vi "FPGAcode4_Debug.vi"() -> ()   [LabVIEW 2015]
uses:
  Limits_In.ctl
  Discard_Points.ctl
  Filter_Cluster.ctl
  <vilib>/Platform/TimedLoop/XDataNode/timing_clust.ctl
  <vilib>/Platform/TimedLoop/XDataNode/nitl_modes.ctl
  <vilib>/Platform/TimedLoop/XDataNode/wakeup.ctl
  Detector_Cluster.ctl
  Correlations.ctl
  <vilib>/rvi/Emulation/niFpgaGetClockAttributes.vi
  <vilib>/rvi/Emulation/niFpgaSctlEmulationGetInTimedLoop.vi
  <vilib>/rvi/Emulation/niFpgaEmulationReportErrorSimple.vi
  <vilib>/rvi/Emulation/niFpgaProcessEmulError.vi
  <vilib>/rvi/eio/common/nirviEmuTemplateMethod_errors.vi
  <vilib>/rvi/Emulation/niFpgaCriticalErrorInLSC.vi
  <vilib>/eio/EIONode/EIONode.xnode
  <vilib>/Platform/TimedLoop/XDataNode/XDataNode.xnode
  <vilib>/Platform/TimedLoop/XDataNode/XDNodeRunTimeDep.lvlib
panel:
  in  "User Trigger?":bool
  out "Charge":T1
  out "Mass":T2
  out "Velocity Count":T3
  in  "User Trigger Distance":fxp<+/-,34,18> format="%.3g"
  out "User Trigger":bool
  out "Particles Discarded":i16
  out "All Discard Points":T4
  in  "Boxcar 3 Size Factor":fxp<+/-,32,16>=0.1999969482421875 format="%.2g"
  in  "Charge Error Factor":fxp<+/-,32,16>=1.100006103515625 format="%.2g"
  in  "Max Correlation Factor":fxp<+,32,4>=0.25 format="%.3g"
  in  "Threshold Factor":fxp<+/-,32,16>=1.0 format="%.2g"
  out "DCS 2":bool
  out "Detectors":cluster{"Det 1":i16, "Det 3":i16}
  out "DCS 1":bool
  in  "Limits":T6
  in  "Calibrate":bool=TRUE
  in  "Armed":bool
  out "Plates":bool
  in  "One Shot":bool
  # "These factors above are in the front\npanel so it is possible to experiment\nwith many different configurations\nof the FPGA on the fly. One can even\nchange the relative size of one filter."
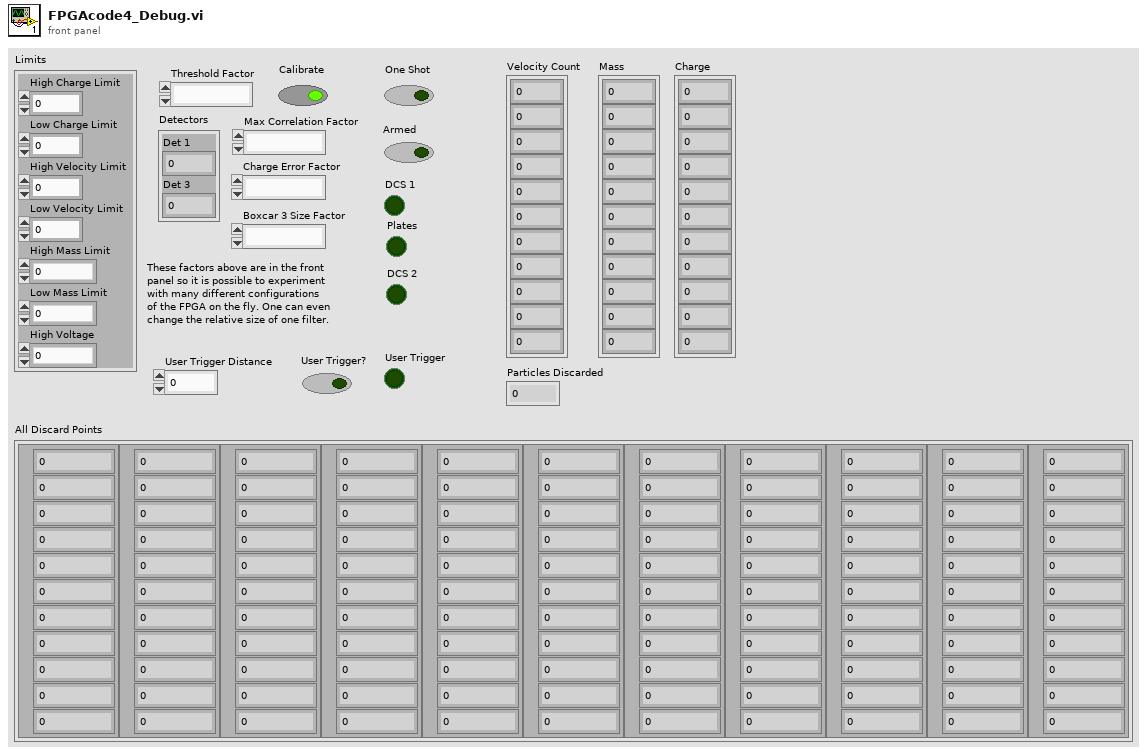
[diagram p1: front panel]
types:
  T1 = cluster{"[0]":fxp<+/-,64,-10>, "[1]":fxp<+/-,64,-10>, "[2]":fxp<+/-,64,-10>, "[3]":fxp<+/-,64,-10>, "[4]":fxp<+/-,64,-10>, "[5]":fxp<+/-,64,-10>, "[6]":fxp<+/-,64,-10>, "[7]":fxp<+/-,64,-10>, "[8]":fxp<+/-,64,-10>, "[9]":fxp<+/-,64,-10>, "[10]":fxp<+/-,64,-10>}
  T2 = cluster{"[0]":fxp<+/-,64,-2>, "[1]":fxp<+/-,64,-2>, "[2]":fxp<+/-,64,-2>, "[3]":fxp<+/-,64,-2>, "[4]":fxp<+/-,64,-2>, "[5]":fxp<+/-,64,-2>, "[6]":fxp<+/-,64,-2>, "[7]":fxp<+/-,64,-2>, "[8]":fxp<+/-,64,-2>, "[9]":fxp<+/-,64,-2>, "[10]":fxp<+/-,64,-2>}
  T3 = cluster{"[0]":i32, "[1]":i32, "[2]":i32, "[3]":i32, "[4]":i32, "[5]":i32, "[6]":i32, "[7]":i32, "[8]":i32, "[9]":i32, "[10]":i32}
  T4 = typedef "Discard_Points.ctl" = cluster{"Discard Points 1":T5, "Discard Points 2":T5, "Discard Points 3":T5, "Discard Points 4":T5, "Discard Points 5":T5, "Discard Points 6":T5, "Discard Points 7":T5, "Discard Points 8":T5, "Discard Points 9":T5, "Discard Points 10":T5, "Discard Points 11":T5}
  T5 = typedef "Filter_Cluster.ctl" = cluster{"1":i32, "2":i32, "3":i32, "4":i32, "5":i32, "6":i32, "7":i32, "8":i32, "9":i32, "10":i32, "11":i32}
  T6 = typedef "Limits_In.ctl" = cluster{"High Charge Limit":fxp<+,32,-41>, "Low Charge Limit":fxp<+,32,-41>, "High Velocity Limit":fxp<+,18,18>, "Low Velocity Limit":fxp<+,18,18>, "High Mass Limit":fxp<+/-,33,-35>, "Low Mass Limit":fxp<+/-,33,-35>, "High Voltage":fxp<+,16,22>}
  T7 = typedef "Detector_Cluster.ctl" = cluster{"Det 1":i32, "Det 2":i32}
  T8 = cluster{"Filter 1":T7, "Filter 2":T7, "Filter 3":T7, "Filter 4":T7}
  T9 = cluster{"Distance to PSU":fxp<+/-,32,5>, "Distance to end of PSU":fxp<+/-,32,5>, "Distance to DCS 2":fxp<+/-,32,5>, "Distance to DCS 1":fxp<+/-,32,5>, "Distance to front of LEIL Chamber":fxp<+/-,32,5>}
  T10 = cluster{"Detector Max Speed Count":i32, "Detector Min Speed Count":i32, "Gap Max Speed Count":i32, "Gap Min Speed Count":i32}
  T11 = cluster{"Distance to PSU":fxp<+/-,64,22>, "Distance to end of PSU":fxp<+/-,64,22>, "Distance to DCS 2":fxp<+/-,64,22>, "Distance to DCS 1":fxp<+/-,64,22>, "Distance to front of LEIL Chamber":fxp<+/-,64,22>}
  T12 = typedef "XDNodeRunTimeDep.lvlib/timing_clust.ctl" = cluster{"Expected End [f-1]":u64, "Actual End [f-1]":u64, "Finished Late? [f-1]":bool, "Expected End [i-1]":u64, "Actual End [i-1]":u64, "Finished Late? [i-1]":bool, "Expected Start [i]":u64, "Actual Start [i]":u64, "Expected Start [f]":u64, "Actual Start [f]":u64, "Source Name":string, "Structure Name":string, "Period":i64, "Deadline":i64, "Offset":i64, "Start":i64, "Priority":i32, "Timeout":i32, "Mode":T13, "Wakeup Reason":T14, "Error":errorcluster, "Source Type":string, "Secondary Source Type":string, "Global End Time":u64, "Global Start Time":u64, "Frame Duration":u64, "Iteration Duration":u64, "Assigned CPU":i32, "I/O Scan Engine Mode":u32}
  T13 = typedef "XDNodeRunTimeDep.lvlib/nitl_modes.ctl" = enum32{"No Change", "Process missed periods, maintain original phase", "Discard missed periods, maintain original phase", "Process missed periods, ignore original phase", "Discard missed periods, ignore original phase"}
  T14 = typedef "XDNodeRunTimeDep.lvlib/wakeup.ctl" = enum32{"Normal", "Aborted", "Asynchronous wakeup", "Timing source error", "Timed loop error", "Timeout"}
  T15 = cluster{"Filter 1":T7, "Filter 2":T7, "Filter 3":T7, "Filter 4":T7}[]
  T16 = cluster{"First Detector Count":i32, "Detector Gap Count":i32, "Second Detector Count":i32, "Second Detector Final Count":i32}
  T17 = typedef "Correlations.ctl" = cluster{"First Correlation":i32, "Latest Correlation":i32}
  T18 = cluster{"Detectors":cluster{"Det 1":i16, "Det 3":i16}, cluster{"Det 1":i16, "Det 2":i16}, cluster{"Det 1":i16, "Det 2":i16}, cluster{"Det 1":i16, "Det 2":i16}}
  T19 = cluster{cluster{"Det 1":i16, "Det 2":i16}, cluster{"Det 1":i16, "Det 2":i16}, cluster{"Det 1":i16, "Det 2":i16}, cluster{"Det 1":i16, "Det 2":i16}}
  T20 = cluster{"Distance to PSU":fxp<+/-,64,54>, "Distance to end of PSU":fxp<+/-,64,54>, "Distance to DCS 2":fxp<+/-,64,54>, "Distance to DCS 1":fxp<+/-,64,54>, "Distance to front of LEIL Chamber":fxp<+/-,64,54>}
  T21 = cluster{"Distance to PSU":i32, "Distance to end of PSU":i32, "Distance to DCS 2":i32, "Distance to DCS 1":i32, "Distance to front of LEIL Chamber":i32}
  T22 = cluster{"[0]":u8, "[1]":u8, "[2]":u8, "[3]":u8, "[4]":u8, "[5]":u8, "[6]":u8, "[7]":u8, "[8]":u8, "[9]":u8, "[10]":u8}
  T23 = cluster{"All Discard Points[0]":T5, "All Discard Points[1]":T5, "All Discard Points[2]":T5, "All Discard Points[3]":T5, "All Discard Points[4]":T5, "All Discard Points[5]":T5, "All Discard Points[6]":T5, "All Discard Points[7]":T5, "All Discard Points[8]":T5, "All Discard Points[9]":T5, "All Discard Points[10]":T5}
  T24 = cluster{i32[], fxp<+/-,64,-2>[], fxp<+/-,64,-10>[]}
  T25 = cluster{"IO Module\\AI 0":i16, "IO Module\\AI 1":i16}
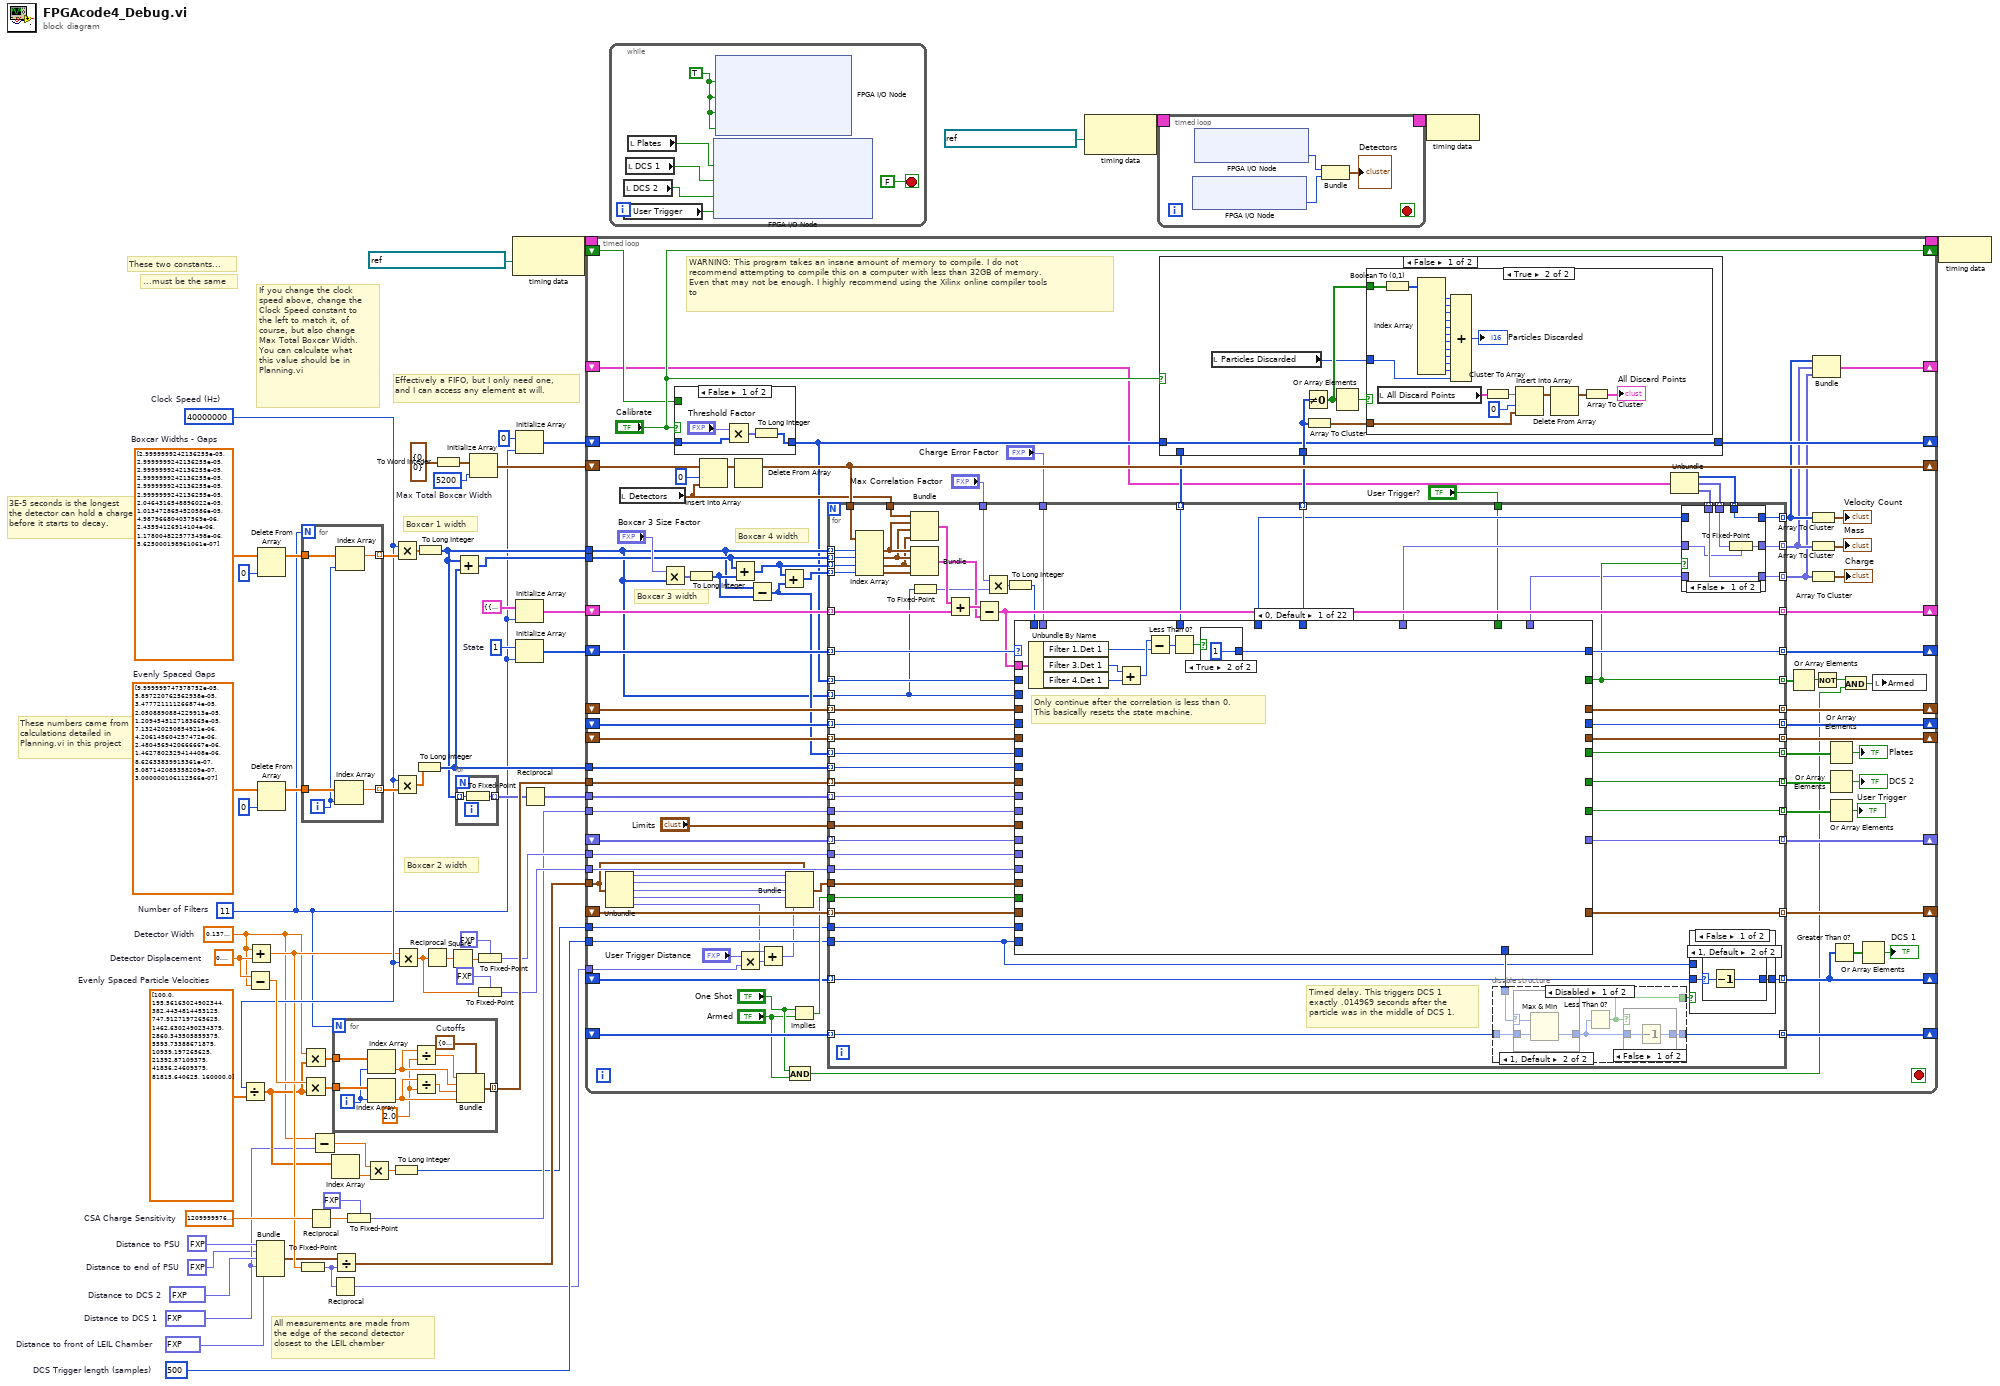
[diagram p0: block diagram]
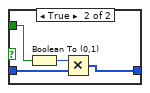
[diagram p2: hidden frame]
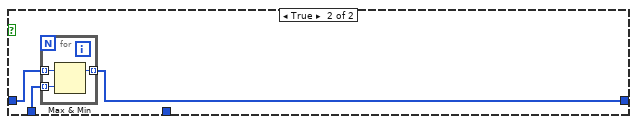
[diagram p4: hidden frame]
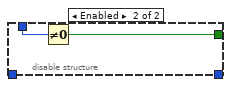
[diagram p10: hidden frame]
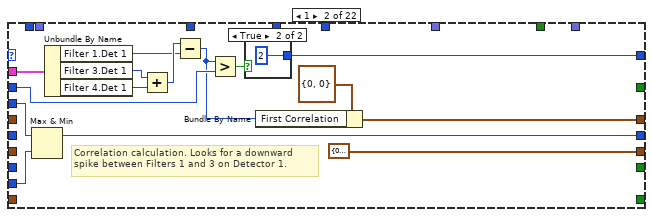
[diagram p12: hidden frame]
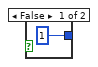
[diagram p13: hidden frame]
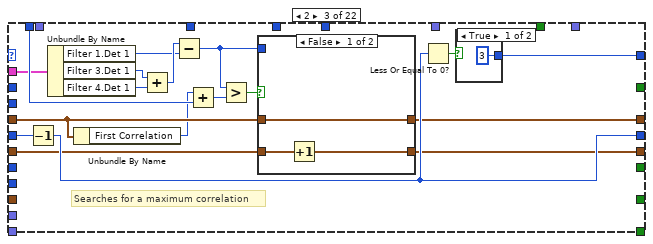
[diagram p14: hidden frame]
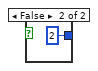
[diagram p15: hidden frame]
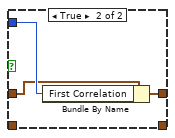
[diagram p16: hidden frame]
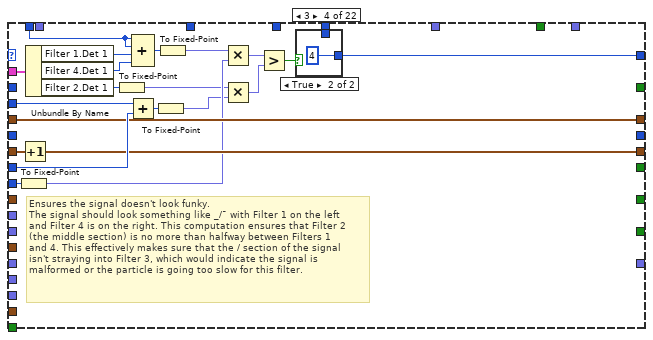
[diagram p17: hidden frame]
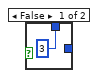
[diagram p18: hidden frame]
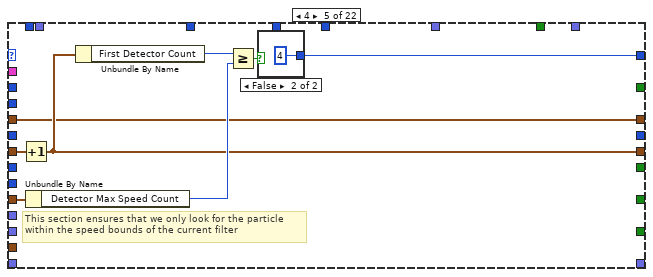
[diagram p19: hidden frame]
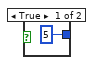
[diagram p20: hidden frame]
diagram:
  w1 = fxp<+/-,32,5> 4.297679997980595  # Distance to front of LEIL Chamber
  w7 = u16 500  # DCS Trigger length (samples)
  w12 = fxp<+/-,32,5> -1.3589000031352043  # Distance to DCS 1
  w16 = fxp<+/-,32,5> 2.6162000000476837  # Distance to DCS 2
  w4 = fxp<+/-,32,5> 1.8999999985098839  # Distance to end of PSU
  w17 = fxp<+/-,32,5> 1.5  # Distance to PSU
  w30 = sgl 12100000000000.0  # CSA Charge Sensitivity
  w52 = u8 1  # State
  w13 = sgl 0.6  # Detector Displacement
  w58 = sgl[] [3e-05, 3e-05, 3e-05, 3e-05, 3e-05, 3e-05, 2.0464317e-05, 1.0134729e-05, 4.987967e-06, 2.4359413e-06, 1.1780048e-06, 5.625e-07]  # Boxcar Widths - Gaps
  w56 = sgl[] [0.0001, 5.8972208e-05, 3.477721e-05, 2.050889e-05, 1.2094545e-05, 7.1324203e-06, 4.2061456e-06, 2.480457e-06, 1.4627802e-06, 8.6263384e-07, 5.087142e-07, 3e-07]  # Evenly Spaced Gaps
  w36 = sgl[] [100.0, 195.56163, 382.44348, 747.9127, 1462.6302, 2860.3435, 5593.734, 10939.197, 21392.871, 41836.246, 81815.64, 160000.0]  # Evenly Spaced Particle Velocities
  w33 = 40000000  # Clock Speed (Hz)
  w8 = sgl 0.138  # Detector Width
  w60 = 5200  # Max Total Boxcar Width
  w5 = 11  # Number of Filters
  # "...must be the same"
  # "These two constants..."
  # "If you change the clock\nspeed above, change the\nClock Speed constant to\nthe left to match it, of\ncourse, but also change\nMax Total Boxcar Width.\nYou can calculate what\nthis value should be in\nPlanning.vi"
  # "All measurements are made from\nthe edge of the second detector\nclosest to the LEIL chamber"
  # "Effectively a FIFO, but I only need one,\nand I can access any element at will."
  # "Boxcar 2 width"
  # "Boxcar 1 width"
  # "3E-5 seconds is the longest\nthe detector can hold a charge\nbefore it starts to decay."
  # "These numbers came from\ncalculations detailed in\nPlanning.vi in this project"
  n1 = Divide(x=w33, y=w36) -> (x/y=w14:sgl[])
  n2 = Subtract(x=w13, y=w8) -> (x-y=w35:sgl)
  n3 = Add(x=w8, y=w13) -> (x+y=w22:sgl)
  n4 = Bundle("Distance to PSU"=w17, "Distance to end of PSU"=w4, "Distance to DCS 2"=w16, "Distance to DCS 1"=w12, "Distance to front of LEIL Chamber"=w1) -> (w21:T9)  [unwired: 1 in]
  n5 = Delete From Array(array=w58, index=0) -> (array with subset deleted=w45:sgl[])  [unwired: 1 in, 1 out]
  n6 = Delete From Array(array=w56, index=0) -> (array with subset deleted=w47:sgl[])  [unwired: 1 in, 1 out]
  n7 = To Fixed-Point(number=w22) -> (fixed-point=w3:fxp<+/-,32,16>)  [unwired: 1 in]
  n8 = for {
    N: w5 -> [_]
    tunnel: w47 -> [w72]
    tunnel: [w69] -> w46 mode=indexing
    tunnel: w45 -> [w71]
    tunnel: [w70] -> w44 mode=indexing
    i -> [w68]
    n9 = Index Array(array=w72, index=w68) -> (element=w69:sgl)
    n10 = Index Array(array=w71, index=w68) -> (element=w70:sgl)
  }
  n11 = Multiply(x=w8, y=w14) -> (x*y=w54:sgl[])
  n12 = Multiply(x=w35, y=w14) -> (x*y=w55:sgl[])
  n13 = Reciprocal(x=w30) -> (1/x=w24:sgl)
  n14 = Subtract(x=w8, y=w12) -> (x-y=w10:sgl)
  n15 = Index Array(array=w14) -> (element=w11:sgl)  [unwired: 1 in]
  n16 = Reciprocal(x=w3) -> (1/x=w2:fxp<+/-,34,18>)
  n17 = for {
    N: w5 -> [_]
    tunnel: w55 -> [w82]
    tunnel: w54 -> [w81]
    tunnel: [w80] -> w49 mode=indexing
    i -> [w79]
    w73 = sgl 2.0 ("y")
    w78 = T10 {"Detector Max Speed Count"=0, "Detector Min Speed Count"=0, "Gap Max Speed Count"=0, "Gap Min Speed Count"=0}  # Cutoffs
    n18 = Index Array(array=w81, index=w79) -> (element=w77:sgl)
    n19 = Index Array(array=w82, index=w79) -> (element=w74:sgl)
    n20 = Divide(x=w77, y=w73) -> (x/y=w76:sgl)
    n21 = Divide(x=w74, y=w73) -> (x/y=w75:sgl)
    n22 = Bundle(cluster=w78, "Detector Max Speed Count"=w76, "Detector Min Speed Count"=w77, "Gap Max Speed Count"=w75, "Gap Min Speed Count"=w74) -> (w80:T10)
  }
  n23 = Divide(x=w21, y=w3) -> (x/y=w20:T11)
  n24 = To Fixed-Point(fixed-point type=fxp<+,32,-43> 0.0, number=w24) -> (fixed-point=w23:fxp<+,32,-43>)
  n25 = Multiply(x=w10, y=w11) -> (x*y=w9:sgl)
  n26 = To Long Integer(number=w9) -> (32bit integer=w6:i32)
  n27 = Multiply(x=w33, y=w44) -> (x*y=w48:sgl[])
  n28 = Multiply(x=w33, y=w46) -> (x*y=w53:sgl[])
  n29 = Multiply(x=w22, y=w33) -> (x*y=w27:sgl)
  n30 = To Long Integer(number=w53) -> (32bit integer=w43:i32[])
  n31 = To Long Integer(number=w48) -> (32bit integer=w39:i32[])
  n32 = Reciprocal(x=w27) -> (1/x=w32:sgl)
  n33 = To Word Integer(number=T7 {"Det 1"=0, "Det 2"=0} ("Detectors")) -> (16bit integer=w42:cluster{"Det 1":i16, "Det 2":i16})
  n34 = Square(x=w32) -> (x^2=w31:sgl)
  n35 = Add(x=w39, y=w43) -> (x+y=w15:i32[])
  n36 = for {
    tunnel: w39 -> [w84] mode=indexing
    tunnel: [w83] -> w38 mode=indexing
    n37 = To Fixed-Point(number=w84) -> (fixed-point=w83:fxp<+/-,32,32>)  [unwired: 1 in]
  }
  n38 = Initialize Array(w42, w60) -> (w61:cluster{"Det 1":i16, "Det 2":i16}[])
  n39 = To Fixed-Point(fixed-point type=fxp<+/-,32,-45> 0.0, number=w31) -> (fixed-point=w34:fxp<+/-,32,-45>)
  n40 = To Fixed-Point(fixed-point type=fxp<+,32,32> 0.0, number=w27) -> (fixed-point=w25:fxp<+,32,32>)
  n41 = node-c288(refnum<k21> "40 MHz Onboard Clock" ("Source Name")) -> (w64:T12)
  n42 = Initialize Array(0 ("element"), w5) -> (w18:i32[])
  n43 = Initialize Array(T8 {"Filter 1"={"Det 1"=0, "Det 2"=0}, "Filter 2"={"Det 1"=0, "Det 2"=0}, "Filter 3"={"Det 1"=0, "Det 2"=0}, "Filter 4"={"Det 1"=0, "Det 2"=0}} ("cluster"), w5) -> (w50:T15)
  n44 = Initialize Array(w52, w5) -> (w51:u8[])
  n45 = Reciprocal(x=w38) -> (1/x=w37:fxp<+/-,34,2>[])
  n46 = timed-loop {
    timing: w64 -> [_]
    timing-out: [_] -> w63
    shift-right: [w169] -> _
    shift-left: w61 -> [w172]
    shift-right: [w168] -> _
    shift-left: w50 -> [w161]
    shift-right: [w166] -> _
    shift-left: w51 -> [w167]
    shift-right: [w165] -> _
    shift-left: _ -> [w164]
    shift-right: [w163] -> _
    shift-left: _ -> [w162]
    tunnel: w49 -> [w159]
    shift-right: [w158] -> _
    shift-left: _ -> [w157]
    tunnel: w39 -> [w146]
    tunnel: w15 -> [w152]
    tunnel: w43 -> [w147]
    tunnel: w37 -> [w145]
    shift-right: [w143] -> _
    shift-left: _ -> [w142]
    tunnel: w34 -> [w141]
    tunnel: w23 -> [w140]
    tunnel: w25 -> [w139]
    tunnel: w20 -> [w117]
    shift-right: [w138] -> _
    shift-left: _ -> [w137]
    shift-right: [w135] -> _
    shift-left: w18 -> [w133]
    shift-right: ["Calibrate"] -> _
    shift-left: _ -> [w130]
    tunnel: w7 -> [w128]
    tunnel: w6 -> [w127]
    shift-right: [w124] -> _
    shift-left: _ -> [w126]
    shift-right: [w122] -> _
    shift-left: _ -> [w121]
    tunnel: w2 -> [w120]
    shift-right: [w91] -> _
    shift-left: _ -> [w90]
    stop <- _ stop-if-true
    # "WARNING: This program takes an insane amount of memory to compile. I do not\nrecommend attempting to compile this on a computer with less than 32GB of memory.\nEven that may not be enough. I highly recommend using the Xilinx online compiler tools\nto"
    # "Boxcar 3 width"
    # "Boxcar 4 width"
    n47 = Unbundle(w117) -> ("Distance to PSU"=w118:fxp<+/-,64,22>, "Distance to end of PSU"=w116:fxp<+/-,64,22>, "Distance to DCS 2"=w115:fxp<+/-,64,22>, "Distance to DCS 1"=w112:fxp<+/-,64,22>, "Distance to front of LEIL Chamber"=w111:fxp<+/-,64,22>)
    n48 = local read "Detectors"() -> (w160:cluster{"Det 1":i16, "Det 3":i16})
    n49 = Multiply(x="Boxcar 3 Size Factor", y=w146) -> (x*y=w154:fxp<+/-,64,48>[])
    n50 = case shown="False" "Calibrate" {
      tunnel: w133 -> [w174 w180]
      tunnel: [w173 w178] -> w132
      tunnel: w130 -> [_ w179]
      frame False {
        n51 = Multiply(x="Threshold Factor", y=w174) -> (x*y=w175:fxp<+/-,64,48>[])
        n52 = To Long Integer(number=w175) -> (32bit integer=w173:i32[])
      }
      frame True {
        n53 = Boolean To (0,1)(Boolean=w179) -> (0, 1=w177:i16)
        n54 = Multiply(x=w177, y=w180) -> (x*y=w178:i32[])
      }
    }
    n55 = To Long Integer(number=w154) -> (32bit integer=w155:i32[])
    n56 = Insert Into Array(array=w172, index=0, new element=w160) -> (w171:cluster{"Det 1":i16, "Det 2":i16}[])
    n57 = Add(x=w152, y=w155) -> (x+y=w151:i32[])
    n58 = Delete From Array(array=w171) -> (array with subset deleted=w169:cluster{"Det 1":i16, "Det 2":i16}[])  [unwired: 2 in, 1 out]
    n59 = Multiply(x="User Trigger Distance", y=w120) -> (x*y=w113:fxp<+/-,64,34>)
    n60 = Subtract(x=w146, y=w155) -> (x-y=w149:i32[])
    n61 = Add(x=w111, y=w113) -> (x+y=w110:fxp<+/-,64,35>)
    n62 = Add(x=w151, y=w149) -> (x+y=w150:i32[])
    n63 = Bundle(cluster=w117, "Distance to PSU"=w118, "Distance to end of PSU"=w116, "Distance to DCS 2"=w115, "Distance to DCS 1"=w112, "Distance to front of LEIL Chamber"=w110) -> (w114:T11)
    n64 = And(x="One Shot", y="Armed") -> (x .and. y?=w100:bool)
    n65 = Implies(1:"Armed", 2:"One Shot") -> (0:w129:bool)
    n66 = Unbundle(w90) -> (w89:i32[], w88:fxp<+/-,64,-2>[], w87:fxp<+/-,64,-10>[])
    n67 = for {
      tunnel: w169 -> [w282]
      tunnel: [w265] -> w168 mode=indexing
      tunnel: w167 -> [w281] mode=indexing
      tunnel: [w279] -> w166 mode=indexing
      tunnel: w132 -> [w280] mode=indexing
      tunnel: [w278] -> w165 mode=indexing
      tunnel: w164 -> [w277] mode=indexing
      tunnel: [w276] -> w163 mode=indexing
      tunnel: w162 -> [w275] mode=indexing
      tunnel: w161 -> [w269] mode=indexing
      tunnel: w160 -> [w274]
      tunnel: w159 -> [w264] mode=indexing
      tunnel: [w263] -> w158 mode=indexing
      tunnel: w157 -> [w262] mode=indexing
      tunnel: w146 -> [w261] mode=indexing
      tunnel: w152 -> [w260] mode=indexing
      tunnel: w151 -> [w259] mode=indexing
      tunnel: w150 -> [w258] mode=indexing
      tunnel: w146 -> [w218] mode=indexing
      tunnel: "Max Correlation Factor" -> [w257]
      tunnel: w149 -> [w256] mode=indexing
      tunnel: w147 -> [w255] mode=indexing
      tunnel: "Charge Error Factor" -> [w254]
      tunnel: [w253] -> w136 mode=indexing
      tunnel: w145 -> [w252] mode=indexing
      tunnel: "Limits" -> [w251]
      tunnel: [w250] -> w143 mode=indexing
      tunnel: w142 -> [w249] mode=indexing
      tunnel: w141 -> [w248]
      tunnel: w140 -> [w247]
      tunnel: w139 -> [w246]
      tunnel: w114 -> [w245]
      tunnel: [w244] -> w138 mode=indexing
      tunnel: w137 -> [w243] mode=indexing
      tunnel: [w242] -> w134 mode=indexing
      tunnel: w129 -> [w241]
      tunnel: w128 -> [w238]
      tunnel: w127 -> [w240]
      tunnel: [w237] -> w124 mode=indexing
      tunnel: w126 -> [w236] mode=indexing
      tunnel: [w234] -> w122 mode=indexing
      tunnel: w121 -> [w233] mode=indexing
      tunnel: [w232] -> w109 mode=indexing
      tunnel: [w231] -> w107 mode=indexing
      tunnel: [w230] -> w106 mode=indexing
      tunnel: [w229] -> w103 mode=indexing
      tunnel: [w223] -> w94 mode=indexing
      tunnel: [w228] -> w92 mode=indexing
      tunnel: [w226] -> w93 mode=indexing
      tunnel: w89 -> [w222] mode=indexing
      tunnel: w88 -> [w221] mode=indexing
      tunnel: w87 -> [w220] mode=indexing
      tunnel: "User Trigger?" -> [w215]
      # "Timed delay. This triggers DCS 1\nexactly .014969 seconds after the\nparticle was in the middle of DCS 1."
      n68 = Index Array(array=w282, index #1=w261, index #2=w260, index #3=w259, index #4=w258) -> (element #1=w272:cluster{"Det 1":i16, "Det 2":i16}, element #2=w271:cluster{"Det 1":i16, "Det 2":i16}, element #3=w270:cluster{"Det 1":i16, "Det 2":i16}, element #4=w273:cluster{"Det 1":i16, "Det 2":i16})
      n69 = Bundle("Detectors"=w274, w272, w271, w270) -> (w268:T18)  [unwired: 1 in]
      n70 = Bundle(w272, w271, w270, w273) -> (w266:T19)  [unwired: 1 in]
      n71 = To Fixed-Point(number=w218) -> (fixed-point=w217:fxp<+/-,32,32>)  [unwired: 1 in]
      n72 = Add(x=w268, y=w269) -> (x+y=w267:T8)
      n73 = Subtract(x=w267, y=w266) -> (x-y=w265:T8)
      n74 = Multiply(x=w257, y=w217) -> (x*y=w219:fxp<+/-,64,36>)
      n75 = To Long Integer(number=w219) -> (32bit integer=w216:i32)
      n76 = case shown="0, Default" w281 {
        tunnel: w280 -> [_ w333 _ _ _ _ _ _ _ _ _ _ _ _ _ _ _ _ _ _ _ _]
        tunnel: [w316 w331 w349 w381 w388 w402 w454 w489 w505 w523 w576 w603 w619 w672 w713 u8 16 ("Det 3") w753 w761 w768 w782 w788 w801] -> w279
        tunnel: w218 -> [_ w322 _ w379 _ w405 _ _ _ w526 _ _ w622 _ _ w743 _ _ _ _ _ _]
        tunnel: [_ w324 w345 w380 w386 w399 w452 w484 w511 w520 w574 w609 w616 w670 _ _ _ _ _ _ _ _] -> w278
        tunnel: w277 -> [_ _ w344 w380 w386 w401 w451 w483 w511 w522 w573 w609 w618 w669 w705 _ _ _ _ _ _ _]
        tunnel: [_ w321 w351 _ _ w403 w456 _ _ w524 w578 _ w620 w674 _ _ _ _ _ _ _ _] -> w276
        tunnel: w275 -> [_ _ w353 _ _ _ w458 _ _ _ w580 _ _ w676 _ _ _ _ _ _ _ _]
        tunnel: w265 -> [w311 w328 w342 w375 _ w406 w449 _ _ w527 w571 _ w623 w667 _ _ _ _ _ _ _ _]
        tunnel: w264 -> [_ _ _ _ w393 w411 w442 _ w510 w532 w564 w608 w628 w660 _ _ _ _ _ _ _ _]
        tunnel: [_ T16 {"First Detector Count"=0, "Detector Gap Count"=0, "Second Detector Count"=0, "Second Detector Final Count"=0} ("Cutoffs") w338 w377 w387 w397 w446 w487 w509 w518 w568 w607 w614 w664 w731 _ _ _ _ _ _ _] -> w263
        tunnel: w262 -> [_ _ w350 w378 w392 w412 w455 w488 w512 w533 w577 w610 w629 w673 w732 w751 _ _ _ _ _ _]
        tunnel: w216 -> [_ _ w352 w362 _ _ w457 _ _ _ w579 _ _ w675 _ _ _ _ _ _ _ _]
        tunnel: w256 -> [_ _ _ w382 _ _ _ _ _ _ _ _ _ _ _ _ _ _ _ _ _ _]
        tunnel: w255 -> [_ w320 _ w370 _ w404 _ _ _ w525 _ _ w621 _ _ _ _ _ _ _ _ _]
        tunnel: w254 -> [_ _ _ _ _ w407 w434 _ _ w528 w556 _ w624 w652 _ _ _ _ _ _ _ _]
        tunnel: [_ _ _ w376 _ w408 w436 w490 _ w529 w558 _ w625 w654 w712 _ _ _ _ _ _ _] -> w253
        tunnel: w252 -> [_ _ _ _ _ _ _ w496 _ _ _ _ _ _ _ _ _ _ _ _ _ _]
        tunnel: w251 -> [_ _ _ _ _ _ _ w501 _ _ _ _ _ _ w733 _ _ _ _ _ _ _]
        tunnel: [_ _ _ _ _ _ _ w480 w504 w515 w554 w602 w613 w650 _ _ _ _ _ _ _ _] -> w250
        tunnel: w249 -> [_ _ _ _ _ _ _ _ w504 w515 w554 w602 w613 w650 w700 _ _ _ _ _ _ _]
        tunnel: w248 -> [_ _ _ _ _ _ _ _ _ _ _ _ _ _ w726 _ _ _ _ _ _ _]
        tunnel: w247 -> [_ _ _ _ _ _ _ w481 _ _ _ _ _ _ _ _ _ _ _ _ _ _]
        tunnel: w246 -> [_ _ _ _ _ _ _ _ _ _ _ _ _ _ w706 _ _ _ _ _ _ _]
        tunnel: w245 -> [_ _ _ _ _ _ _ _ _ _ _ _ _ _ _ w747 _ _ _ _ _ _]
        tunnel: [_ _ _ _ _ _ _ _ _ _ _ _ _ _ _ w739 w755 w763 w770 w779 w790 w799] -> w244
        tunnel: w243 -> [_ _ _ _ _ _ _ _ _ _ _ _ _ _ _ _ w756 w764 w771 w780 w791 w800]
        tunnel: [_ _ _ _ _ _ _ _ _ _ _ _ _ _ w704 _ _ _ _ _ _ _] -> w242
        tunnel: w241 -> [_ _ _ _ _ _ _ _ _ _ _ _ _ _ w703 _ _ _ _ _ _ _]
        tunnel: w240 -> [_ _ _ _ _ _ _ _ _ _ _ _ _ _ _ w738 _ _ _ _ _ _]
        tunnel: w238 -> [_ _ _ _ _ _ _ _ _ _ _ _ _ _ _ _ _ _ _ w777 _ w797]
        tunnel: [_ _ _ _ _ _ _ _ _ _ _ _ _ _ _ w736 _ _ _ _ _ _] -> w239
        tunnel: [_ _ _ _ _ _ _ _ _ _ _ _ _ _ _ _ _ TRUE _ _ _ _] -> w232
        tunnel: [_ _ _ _ _ _ _ _ _ _ _ _ _ _ _ _ _ _ _ TRUE _ _] -> w231
        tunnel: [_ _ _ _ _ _ _ _ _ _ _ _ _ _ _ _ _ _ _ _ _ TRUE] -> w230
        tunnel: [_ _ _ _ _ _ _ _ _ _ _ _ _ _ w702 _ _ _ _ _ _ _] -> w229
        tunnel: [_ _ _ _ _ _ _ _ _ _ _ _ _ _ w701 _ _ _ _ _ _ _] -> w224
        tunnel: [_ _ _ _ _ _ _ _ _ _ _ _ _ _ w700 _ _ _ _ _ _ _] -> w227
        tunnel: [_ _ _ _ _ _ _ _ _ _ _ _ _ _ w699 _ _ _ _ _ _ _] -> w225
        tunnel: w215 -> [_ _ _ _ _ _ _ _ _ _ _ _ _ _ _ _ _ _ _ w774 _ _]
        frame 0, Default {
          # "Only continue after the correlation is less than 0.\nThis basically resets the state machine."
          n77 = Unbundle By Name(w311) -> ("Filter 1.Det 1"=w312:i32, "Filter 3.Det 1"=w313:i32, "Filter 4.Det 1"=w314:i32)
          n78 = Add(x=w313, y=w314) -> (x+y=w315:i32)
          n79 = Subtract(x=w315, y=w312) -> (x-y=w310:i32)
          n80 = Less Than 0?(x=w310) -> (x < 0?=w317:bool)
          n81 = case shown="True" w317 {
            tunnel: [_ u8 1 ("Det 3")] -> w316
            frame False {
            }
            frame True {
            }
          }
        }
        frame 1 {
          # "Correlation calculation. Looks for a downward\nspike between Filters 1 and 3 on Detector 1."
          n82 = Max & Min(x=w322, y=w320) -> (max(x,y)=w321:i32)  [unwired: 1 out]
          n83 = Unbundle By Name(w328) -> ("Filter 1.Det 1"=w325:i32, "Filter 3.Det 1"=w326:i32, "Filter 4.Det 1"=w327:i32)
          n84 = Add(x=w326, y=w327) -> (x+y=w329:i32)
          n85 = Subtract(x=w329, y=w325) -> (x-y=w330:i32)
          n86 = Greater?(x=w330, y=w333) -> (0:w332:bool)
          n87 = case shown="True" w332 {
            tunnel: [u8 1 ("Det 3") u8 2 ("Det 3")] -> w331
            frame False {
            }
            frame True {
            }
          }
          n88 = Bundle By Name(cluster=T17 {"First Correlation"=0, "Latest Correlation"=0}, "First Correlation"=w330) -> (w324:T17)
        }
        frame 2 {
          # "Searches for a maximum correlation"
          n89 = Decrement(x=w353) -> (x-1=w351:i32)
          n90 = Unbundle By Name(w342) -> ("Filter 1.Det 1"=w341:i32, "Filter 3.Det 1"=w340:i32, "Filter 4.Det 1"=w339:i32)
          n91 = Unbundle By Name(w344) -> ("First Correlation"=w336:i32)
          n92 = Add(x=w340, y=w339) -> (x+y=w348:i32)
          n93 = Subtract(x=w348, y=w341) -> (x-y=w343:i32)
          n94 = Add(x=w336, y=w352) -> (x+y=w337:i32)
          n95 = Greater?(x=w343, y=w337) -> (0:w347:bool)
          n96 = case shown="False" w347 {
            tunnel: [w356 _] -> w338
            tunnel: w350 -> [w357 _]
            tunnel: w343 -> [_ w361]
            tunnel: [w358 w360] -> w345
            tunnel: w344 -> [w358 w359]
            frame False {
              n97 = Increment(x=w357) -> (x+1=w356:T16)
            }
            frame True {
              n98 = Bundle By Name(cluster=w359, "First Correlation"=w361) -> (w360:T17)
            }
          }
          n99 = Less Or Equal To 0?(x=w351) -> (x <= 0?=w346:bool)
          n100 = case shown="True" w346 {
            tunnel: [u8 3 ("Det 3") u8 2 ("Det 3")] -> w349
            frame True {
            }
            frame False {
            }
          }
        }
        frame 3 {
          # "Ensures the signal doesn't look funky.\nThe signal should look something like _/¯ with Filter 1 on the left\nand Filter 4 is on the right. This computation ensures that Filter 2\n(the middle section) is no more than halfway between Filters 1\nand 4. This effectively makes sure that the / section of the signal\nisn't straying into Filter 3, which would indicate the signal is\nmalformed or the particle is going too slow for this filter."
          n101 = To Fixed-Point(number=w370) -> (fixed-point=w368:fxp<+/-,32,32>)  [unwired: 1 in]
          n102 = Increment(x=w378) -> (x+1=w377:T16)
          n103 = Unbundle By Name(w375) -> ("Filter 1.Det 1"=w373:i32, "Filter 4.Det 1"=w374:i32, "Filter 2.Det 1"=w371:i32)
          n104 = To Fixed-Point(number=w371) -> (fixed-point=w367:fxp<+/-,32,32>)  [unwired: 1 in]
          n105 = Add(x=w379, y=w382) -> (x+y=w372:i32)
          n106 = Compound Arithmetic op=ADD(w362, w362, w373, w374) -> (w383:i32)
          n107 = To Fixed-Point(number=w372) -> (fixed-point=w366:fxp<+/-,32,32>)  [unwired: 1 in]
          n108 = To Fixed-Point(number=w383) -> (fixed-point=w363:fxp<+/-,32,32>)  [unwired: 1 in]
          n109 = Multiply(x=w363, y=w368) -> (x*y=w364:fxp<+/-,64,64>)
          n110 = Multiply(x=w367, y=w366) -> (x*y=w365:fxp<+/-,64,64>)
          n111 = Greater?(x=w364, y=w365) -> (0:w369:bool)
          n112 = case shown="True" w369 {
            tunnel: [_ u8 4] -> w381
            tunnel: [u8 3 _] -> w376
            frame False {
            }
            frame True {
            }
          }
        }
        frame 4 {
          # "This section ensures that we only look for the particle\nwithin the speed bounds of the current filter"
          n113 = Increment(x=w392) -> (x+1=w387:T16)
          n114 = Unbundle By Name(w393) -> ("Detector Max Speed Count"=w390:i32)
          n115 = Unbundle By Name(w387) -> ("First Detector Count"=w391:i32)
          n116 = Greater Or Equal?(x=w391, y=w390) -> (x >= y?=w389:bool)
          n117 = case shown="False" w389 {
            tunnel: [u8 5 u8 4] -> w388
            frame True {
            }
            frame False {
            }
          }
        }
        frame 5 {
          # "Waits for a reverse correlation that's close to the first correlation, but make sure it's in the right speed range."
          n118 = Increment(x=w412) -> (x+1=w396:T16)
          n119 = Unbundle By Name(w411) -> ("Detector Min Speed Count"=w410:i32)
          n120 = Unbundle By Name(w401) -> ("First Correlation"=w400:i32)
          n121 = Unbundle By Name(w396) -> ("First Detector Count"=w398:i32)
          n122 = Greater Or Equal?(x=w398, y=w410) -> (x >= y?=w409:bool)
          n123 = case shown="False" w409 {
            tunnel: [_ w430] -> w402
            tunnel: [u8 5 _] -> w408
            tunnel: w407 -> [_ w429]
            tunnel: w406 -> [_ w426]
            tunnel: w400 -> [_ w416]
            tunnel: [_ w414] -> w399
            frame True {
            }
            frame False {
              n124 = Unbundle By Name(w426) -> ("Filter 1.Det 1"=w423:i32, "Filter 3.Det 1"=w425:i32, "Filter 4.Det 1"=w424:i32)
              n125 = To Fixed-Point(number=w416) -> (fixed-point=w419:fxp<+/-,32,32>)  [unwired: 1 in]
              n126 = Subtract(x=fxp<+,1,2> 2.0, y=w429) -> (x-y=w427:fxp<+/-,33,17>)
              n127 = Add(x=w425, y=w424) -> (x+y=w422:i32)
              n128 = Multiply(x=w427, y=w419) -> (x*y=w421:fxp<+/-,64,48>)
              n129 = Subtract(x=w423, y=w422) -> (x-y=w415:i32)
              n130 = To Fixed-Point(number=w415) -> (fixed-point=w418:fxp<+/-,32,32>)  [unwired: 1 in]
              n131 = Greater?(x=w418, y=w421) -> (0:w420:bool)
              n132 = case shown="False" w420 {
                tunnel: [u8 6 u8 5] -> w430
                frame True {
                }
                frame False {
                }
              }
              n133 = Bundle(cluster=T17 {"First Correlation"=0, "Latest Correlation"=0} ("input cluster"), "First Correlation"=w416, "Latest Correlation"=w415) -> (w414:T17)
            }
          }
          n134 = Max & Min(x=w405, y=w404) -> (max(x,y)=w403:i32)  [unwired: 1 out]
          n135 = Bundle(cluster=w396, "First Detector Count"=w398) -> (w397:T16)  [unwired: 3 in]
        }
        frame 6 {
          # "Searches for a maximum correlation. If the maximum correlation happens\nafter the speed limit, this isn't the right filter, and we go back to the beginning.\nIf the maximum correlation is too big, we also go back to the beginning."
          n136 = Decrement(x=w458) -> (x-1=w456:i32)
          n137 = Unbundle By Name(w449) -> ("Filter 1.Det 1"=w438:i32, "Filter 3.Det 1"=w448:i32, "Filter 4.Det 1"=w447:i32)
          n138 = Unbundle By Name(w442) -> ("Detector Min Speed Count"=w440:i32)
          n139 = Unbundle By Name(w451) -> ("Latest Correlation"=w444:i32)
          n140 = Add(x=w448, y=w447) -> (x+y=w437:i32)
          n141 = Subtract(x=w438, y=w437) -> (x-y=w450:i32)
          n142 = Increment(x=w455) -> (x+1=w443:T16)
          n143 = Add(x=w444, y=w457) -> (x+y=w445:i32)
          n144 = Greater?(x=w450, y=w445) -> (0:w453:bool)
          n145 = case shown="True" w453 {
            tunnel: [w465 w478] -> w446
            tunnel: w443 -> [w465 w475]
            tunnel: w450 -> [_ w469]
            tunnel: [w466 w477] -> w452
            tunnel: w451 -> [w466 w476]
            tunnel: [_ w474] -> w441
            tunnel: w434 -> [_ w473]
            tunnel: [_ w467] -> w433
            frame False {
            }
            frame True {
              n146 = Unbundle(w475) -> ("First Detector Count"=w474:i32)  [unwired: 3 out]
              n147 = Unbundle(w476) -> ("First Correlation"=w472:i32)  [unwired: 1 out]
              n148 = Bundle(cluster=w475, "First Detector Count"=w474) -> (w478:T16)  [unwired: 3 in]
              n149 = To Fixed-Point(number=w472) -> (fixed-point=w471:fxp<+/-,32,32>)  [unwired: 1 in]
              n150 = Bundle(cluster=w476, "First Correlation"=w472, "Latest Correlation"=w469) -> (w477:T17)
              n151 = To Fixed-Point(number=w469) -> (fixed-point=w468:fxp<+/-,32,32>)  [unwired: 1 in]
              n152 = Multiply(x=w473, y=w471) -> (x*y=w470:fxp<+/-,64,48>)
              n153 = Less?(x=w470, y=w468) -> (x < y?=w467:bool)
            }
          }
          n154 = Greater?(x=w441, y=w440) -> (0:w439:bool)
          n155 = Or(x=w433, y=w439) -> (x .or. y?=w435:bool)
          n156 = case shown="False" w435 {
            tunnel: w456 -> [w461 _]
            tunnel: [w460 _] -> w454
            tunnel: [_ u8 6 ("Det 3")] -> w436
            frame False {
              n157 = Less Or Equal To 0?(x=w461) -> (x <= 0?=w459:bool)
              n158 = case shown="True" w459 {
                tunnel: [u8 7 ("Det 3") u8 6 ("Det 3")] -> w460
                frame True {
                }
                frame False {
                }
              }
            }
            frame True {
            }
          }
        }
        frame 7 {
          # "q = integer charge / CSA sensitivity"
          # "Ensures the charge is good"
          n159 = Unbundle(w483) -> ("First Correlation"=w500:i32, "Latest Correlation"=w499:i32)
          n160 = Unbundle By Name(w501) -> ("High Charge Limit"=w495:fxp<+,32,-41>, "Low Charge Limit"=w494:fxp<+,32,-41>)
          n161 = Add(x=w500, y=w499) -> (x+y=w498:i32)
          n162 = To Fixed-Point(number=w498) -> (fixed-point=w497:fxp<+/-,32,32>)  [unwired: 1 in]
          n163 = Scale By Power Of 2(n=i16 -1, x=w497) -> (x*2^n=w486:fxp<+/-,32,32>)
          n164 = Multiply(x=w486, y=w496) -> (x*y=w482:fxp<+/-,64,33>)
          n165 = Increment(x=w488) -> (x+1=w487:T16)
          n166 = To Long Integer(number=w486) -> (32bit integer=w485:i32)
          n167 = Multiply(x=w482, y=w481) -> (x*y=w480:fxp<+/-,64,-10>)
          n168 = Bundle(cluster=w483, "First Correlation"=w485) -> (w484:T17)  [unwired: 1 in]
          n169 = Less?(x=w480, y=w495) -> (x < y?=w493:bool)
          n170 = Greater?(x=w480, y=w494) -> (0:w492:bool)
          n171 = And(x=w493, y=w492) -> (x .and. y?=w491:bool)
          n172 = case shown="False" w491 {
            tunnel: [u8 7 ("Det 3") _] -> w490
            tunnel: [_ u8 8 ("Det 3")] -> w489
            frame True {
            }
            frame False {
            }
          }
        }
        frame 8 {
          # "Wait for the particle to get to the second detector."
          n173 = Increment(x=w512) -> (x+1=w509:T16)
          n174 = Unbundle By Name(w510) -> ("Gap Max Speed Count"=w507:i32)
          n175 = Unbundle By Name(w509) -> ("Detector Gap Count"=w508:i32)
          n176 = Greater Or Equal?(x=w508, y=w507) -> (x >= y?=w506:bool)
          n177 = case shown="True" w506 {
            tunnel: [u8 9 ("State") u8 8 ("State")] -> w505
            frame True {
            }
            frame False {
            }
          }
        }
        frame 9 {
          # "Waits for a correlation that's close to the first two correlations."
          n178 = Increment(x=w533) -> (x+1=w517:T16)
          n179 = Unbundle By Name(w522) -> ("First Correlation"=w521:i32)
          n180 = Unbundle By Name(w532) -> ("Gap Min Speed Count"=w531:i32)
          n181 = Unbundle(w517) -> ("First Detector Count"=w519:i32, "Detector Gap Count"=w516:i32)  [unwired: 2 out]
          n182 = Greater Or Equal?(x=w516, y=w531) -> (x >= y?=w530:bool)
          n183 = case shown="False" w530 {
            tunnel: [_ w551] -> w523
            tunnel: [u8 9 _] -> w529
            tunnel: w528 -> [_ w550]
            tunnel: w527 -> [_ w547]
            tunnel: w521 -> [_ w537]
            tunnel: [_ w535] -> w520
            frame True {
            }
            frame False {
              n184 = Unbundle By Name(w547) -> ("Filter 1.Det 2"=w544:i32, "Filter 3.Det 2"=w546:i32, "Filter 4.Det 2"=w545:i32)
              n185 = To Fixed-Point(number=w537) -> (fixed-point=w540:fxp<+/-,32,32>)  [unwired: 1 in]
              n186 = Subtract(x=fxp<+,1,2> 2.0, y=w550) -> (x-y=w548:fxp<+/-,33,17>)
              n187 = Add(x=w546, y=w545) -> (x+y=w543:i32)
              n188 = Multiply(x=w548, y=w540) -> (x*y=w542:fxp<+/-,64,48>)
              n189 = Subtract(x=w543, y=w544) -> (x-y=w536:i32)
              n190 = To Fixed-Point(number=w536) -> (fixed-point=w539:fxp<+/-,32,32>)  [unwired: 1 in]
              n191 = Greater?(x=w539, y=w542) -> (0:w541:bool)
              n192 = case shown="True" w541 {
                tunnel: [u8 10 u8 9] -> w551
                frame True {
                }
                frame False {
                }
              }
              n193 = Bundle(cluster=T17 {"First Correlation"=0, "Latest Correlation"=0} ("input cluster"), "First Correlation"=w537, "Latest Correlation"=w536) -> (w535:T17)
            }
          }
          n194 = Max & Min(x=w526, y=w525) -> (max(x,y)=w524:i32)  [unwired: 1 out]
          n195 = Bundle(cluster=w517, "First Detector Count"=w519, "Detector Gap Count"=w516) -> (w518:T16)  [unwired: 2 in]
        }
        frame 10 {
          # "Searches for a maximum correlation. If the maximum correlation happens\nafter the speed limit, this isn't the right filter, and we go back to the beginning.\nIf the maximum correlation is too big, we also go back to the beginning."
          n196 = Decrement(x=w580) -> (x-1=w578:i32)
          n197 = Unbundle By Name(w571) -> ("Filter 1.Det 2"=w560:i32, "Filter 3.Det 2"=w570:i32, "Filter 4.Det 2"=w569:i32)
          n198 = Unbundle By Name(w564) -> ("Gap Min Speed Count"=w562:i32)
          n199 = Unbundle By Name(w573) -> ("Latest Correlation"=w566:i32)
          n200 = Add(x=w570, y=w569) -> (x+y=w559:i32)
          n201 = Subtract(x=w559, y=w560) -> (x-y=w572:i32)
          n202 = Increment(x=w577) -> (x+1=w565:T16)
          n203 = Add(x=w566, y=w579) -> (x+y=w567:i32)
          n204 = Greater?(x=w572, y=w567) -> (0:w575:bool)
          n205 = case shown="True" w575 {
            tunnel: [w587 w601] -> w568
            tunnel: w565 -> [w587 w598]
            tunnel: w572 -> [_ w592]
            tunnel: [w588 w600] -> w574
            tunnel: w573 -> [w588 w599]
            tunnel: [_ w589] -> w563
            tunnel: w556 -> [_ w596]
            tunnel: [_ w590] -> w555
            frame False {
            }
            frame True {
              n206 = Unbundle(w598) -> ("First Detector Count"=w597:i32, "Detector Gap Count"=w589:i32)  [unwired: 2 out]
              n207 = Unbundle(w599) -> ("First Correlation"=w595:i32)  [unwired: 1 out]
              n208 = Bundle(cluster=w598, "First Detector Count"=w597, "Detector Gap Count"=w589) -> (w601:T16)  [unwired: 2 in]
              n209 = To Fixed-Point(number=w595) -> (fixed-point=w594:fxp<+/-,32,32>)  [unwired: 1 in]
              n210 = Bundle(cluster=w599, "First Correlation"=w595, "Latest Correlation"=w592) -> (w600:T17)
              n211 = To Fixed-Point(number=w592) -> (fixed-point=w591:fxp<+/-,32,32>)  [unwired: 1 in]
              n212 = Multiply(x=w596, y=w594) -> (x*y=w593:fxp<+/-,64,48>)
              n213 = Less?(x=w593, y=w591) -> (x < y?=w590:bool)
            }
          }
          n214 = Greater?(x=w563, y=w562) -> (0:w561:bool)
          n215 = Or(x=w555, y=w561) -> (x .or. y?=w557:bool)
          n216 = case shown="False" w557 {
            tunnel: w578 -> [w583 _]
            tunnel: [w582 _] -> w576
            tunnel: [_ u8 10 ("Det 3")] -> w558
            frame False {
              n217 = Less Or Equal To 0?(x=w583) -> (x <= 0?=w581:bool)
              n218 = case shown="True" w581 {
                tunnel: [u8 11 ("Det 3") u8 10 ("Det 3")] -> w582
                frame True {
                }
                frame False {
                }
              }
            }
            frame True {
            }
          }
        }
        frame 11 {
          # "Wait for the particle to get to the second detector."
          n219 = Increment(x=w610) -> (x+1=w607:T16)
          n220 = Unbundle By Name(w608) -> ("Detector Max Speed Count"=w605:i32)
          n221 = Unbundle By Name(w607) -> ("Second Detector Count"=w606:i32)
          n222 = Greater Or Equal?(x=w606, y=w605) -> (x >= y?=w604:bool)
          n223 = case shown="True" w604 {
            tunnel: [u8 12 ("State") u8 11 ("State")] -> w603
            frame True {
            }
            frame False {
            }
          }
        }
        frame 12 {
          # "Waits for a reverse correlation that's close to the first two correlations."
          n224 = Increment(x=w629) -> (x+1=w614:T16)
          n225 = Unbundle By Name(w618) -> ("First Correlation"=w617:i32)
          n226 = Unbundle By Name(w628) -> ("Detector Min Speed Count"=w627:i32)
          n227 = Unbundle By Name(w614) -> ("Second Detector Count"=w615:i32)
          n228 = Greater Or Equal?(x=w615, y=w627) -> (x >= y?=w626:bool)
          n229 = case shown="False" w626 {
            tunnel: [_ w647] -> w619
            tunnel: [u8 12 _] -> w625
            tunnel: w624 -> [_ w646]
            tunnel: w623 -> [_ w643]
            tunnel: w617 -> [_ w633]
            tunnel: [_ w631] -> w616
            frame True {
            }
            frame False {
              n230 = Unbundle By Name(w643) -> ("Filter 1.Det 2"=w640:i32, "Filter 3.Det 2"=w642:i32, "Filter 4.Det 2"=w641:i32)
              n231 = To Fixed-Point(number=w633) -> (fixed-point=w636:fxp<+/-,32,32>)  [unwired: 1 in]
              n232 = Subtract(x=fxp<+,1,2> 2.0, y=w646) -> (x-y=w644:fxp<+/-,33,17>)
              n233 = Add(x=w642, y=w641) -> (x+y=w639:i32)
              n234 = Multiply(x=w644, y=w636) -> (x*y=w638:fxp<+/-,64,48>)
              n235 = Subtract(x=w640, y=w639) -> (x-y=w632:i32)
              n236 = To Fixed-Point(number=w632) -> (fixed-point=w635:fxp<+/-,32,32>)  [unwired: 1 in]
              n237 = Greater?(x=w635, y=w638) -> (0:w637:bool)
              n238 = case shown="True" w637 {
                tunnel: [u8 13 u8 12] -> w647
                frame True {
                }
                frame False {
                }
              }
              n239 = Bundle(cluster=T17 {"First Correlation"=0, "Latest Correlation"=0} ("input cluster"), "First Correlation"=w633, "Latest Correlation"=w632) -> (w631:T17)
            }
          }
          n240 = Max & Min(x=w622, y=w621) -> (max(x,y)=w620:i32)  [unwired: 1 out]
        }
        frame 13 {
          # "Searches for a maximum correlation. If the maximum correlation happens\nafter the speed limit, this isn't the right filter, and we go back to the beginning.\nIf the maximum correlation is too big, we also go back to the beginning."
          n241 = Decrement(x=w676) -> (x-1=w674:i32)
          n242 = Unbundle By Name(w667) -> ("Filter 1.Det 2"=w656:i32, "Filter 3.Det 2"=w666:i32, "Filter 4.Det 2"=w665:i32)
          n243 = Unbundle By Name(w660) -> ("Detector Min Speed Count"=w658:i32)
          n244 = Unbundle By Name(w669) -> ("Latest Correlation"=w662:i32)
          n245 = Add(x=w666, y=w665) -> (x+y=w655:i32)
          n246 = Subtract(x=w656, y=w655) -> (x-y=w668:i32)
          n247 = Increment(x=w673) -> (x+1=w661:T16)
          n248 = Add(x=w662, y=w675) -> (x+y=w663:i32)
          n249 = Greater?(x=w668, y=w663) -> (0:w671:bool)
          n250 = case shown="True" w671 {
            tunnel: [w683 w698] -> w664
            tunnel: w661 -> [w683 w695]
            tunnel: w668 -> [_ w689]
            tunnel: [w684 w697] -> w670
            tunnel: w669 -> [w684 w696]
            tunnel: [_ w685] -> w659
            tunnel: w652 -> [_ w693]
            tunnel: [_ w687] -> w651
            frame False {
            }
            frame True {
              n251 = Unbundle(w695) -> ("First Detector Count"=w694:i32, "Detector Gap Count"=w686:i32, "Second Detector Count"=w685:i32)  [unwired: 1 out]
              n252 = Unbundle(w696) -> ("First Correlation"=w692:i32)  [unwired: 1 out]
              n253 = Bundle(cluster=w695, "First Detector Count"=w694, "Detector Gap Count"=w686, "Second Detector Count"=w685) -> (w698:T16)  [unwired: 1 in]
              n254 = To Fixed-Point(number=w692) -> (fixed-point=w691:fxp<+/-,32,32>)  [unwired: 1 in]
              n255 = Bundle(cluster=w696, "First Correlation"=w692, "Latest Correlation"=w689) -> (w697:T17)
              n256 = To Fixed-Point(number=w689) -> (fixed-point=w688:fxp<+/-,32,32>)  [unwired: 1 in]
              n257 = Multiply(x=w693, y=w691) -> (x*y=w690:fxp<+/-,64,48>)
              n258 = Less?(x=w690, y=w688) -> (x < y?=w687:bool)
            }
          }
          n259 = Greater?(x=w659, y=w658) -> (0:w657:bool)
          n260 = Or(x=w651, y=w657) -> (x .or. y?=w653:bool)
          n261 = case shown="False" w653 {
            tunnel: w674 -> [w679 _]
            tunnel: [w678 _] -> w672
            tunnel: [_ u8 13 ("Det 3")] -> w654
            frame False {
              n262 = Less Or Equal To 0?(x=w679) -> (x <= 0?=w677:bool)
              n263 = case shown="True" w677 {
                tunnel: [u8 14 ("Det 3") u8 13 ("Det 3")] -> w678
                frame True {
                }
                frame False {
                }
              }
            }
            frame True {
            }
          }
        }
        frame 14 {
          # "v = clockspeed * distance / speed count"
          # "1/2mv^2 = Vq\ntherefore\nm = 2Vq/v^2"
          n264 = Increment(x=w732) -> (x+1=w731:T16)
          n265 = Unbundle By Name(w733) -> ("High Velocity Limit"=w710:fxp<+,18,18>, "Low Velocity Limit"=w711:fxp<+,18,18>, "High Mass Limit"=w721:fxp<+/-,33,-35>, "Low Mass Limit"=w722:fxp<+/-,33,-35>, "High Voltage"=w716:fxp<+,16,22>)
          n266 = Unbundle By Name(w731) -> ("First Detector Count"=w730:i32, "Second Detector Final Count"=w729:i32)
          n267 = Unbundle By Name(w705) -> ("First Correlation"=w704:i32)
          n268 = Multiply(x=w716, y=w700) -> (x*y=w723:fxp<+/-,64,12>)
          n269 = Subtract(x=w730, y=w729) -> (x-y=w701:i32)
          n270 = Square(x=w701) -> (x^2=w728:i32)
          n271 = To Fixed-Point(number=w701) -> (fixed-point=w709:fxp<+/-,32,32>)  [unwired: 1 in]
          n272 = To Fixed-Point(fixed-point type=fxp<+,32,32> 0.0, number=w728) -> (fixed-point=w725:fxp<+,32,32>)
          n273 = Multiply(x=w710, y=w709) -> (x*y=w708:fxp<+/-,50,50>)
          n274 = Multiply(x=w709, y=w711) -> (x*y=w707:fxp<+/-,50,50>)
          n275 = Scale By Power Of 2(n=i16 1, x=w725) -> (x*2^n=w715:fxp<+,32,32>)
          n276 = Multiply(x=w726, y=w715) -> (x*y=w724:fxp<+/-,64,-13>)
          n277 = Less Or Equal?(x=w708, y=w706) -> (x <= y?=w720:bool)
          n278 = Greater Or Equal?(x=w707, y=w706) -> (x >= y?=w719:bool)
          n279 = Multiply(x=w723, y=w724) -> (x*y=w699:fxp<+/-,64,-2>)
          n280 = Less Or Equal?(x=w699, y=w721) -> (x <= y?=w718:bool)
          n281 = Greater Or Equal?(x=w699, y=w722) -> (x >= y?=w717:bool)
          n282 = Compound Arithmetic op=AND(w720, w719, w718, w717, w703) -> (w702:bool)
          n283 = case shown="True" w702 {
            tunnel: [u8 15 ("Det 3") _] -> w713
            tunnel: [_ u8 14 ("Det 3")] -> w712
            frame True {
            }
            frame False {
            }
          }
        }
        frame 15 {
          n284 = Increment(x=w751) -> (x+1=w750:T16)
          n285 = Unbundle By Name(w750) -> ("First Detector Count"=w749:i32, "Detector Gap Count"=w740:i32)
          n286 = Subtract(x=w749, y=w740) -> (x-y=w746:i32)
          n287 = To Fixed-Point(number=w746) -> (fixed-point=w748:fxp<+/-,32,32>)  [unwired: 1 in]
          n288 = Multiply(x=w748, y=w747) -> (x*y=w745:T20)
          n289 = To Long Integer(number=w745) -> (32bit integer=w744:T21)
          n290 = Subtract(x=w744, y=w743) -> (x-y=w742:T21)
          n291 = Subtract(x=w742, y=w740) -> (x-y=w739:T21)
          n292 = Unbundle By Name(w739) -> ("Distance to DCS 1"=w737:i32)
          n293 = Add(x=w737, y=w738) -> (x+y=w736:i32)
        }
        frame 16 {
          n294 = Decrement(x=w756) -> (x-1=w755:T21)
          n295 = Unbundle By Name(w755) -> ("Distance to PSU"=w754:i32)
          n296 = Less Or Equal To 0?(x=w754) -> (x <= 0?=w752:bool)
          n297 = case shown="True" w752 {
            tunnel: [u8 17 ("Det 3") u8 16 ("Det 3")] -> w753
            frame True {
            }
            frame False {
            }
          }
        }
        frame 17 {
          n298 = Decrement(x=w764) -> (x-1=w763:T21)
          n299 = Unbundle By Name(w763) -> ("Distance to end of PSU"=w762:i32)
          n300 = Less Or Equal To 0?(x=w762) -> (x <= 0?=w760:bool)
          n301 = case shown="True" w760 {
            tunnel: [u8 18 ("Det 3") u8 17 ("Det 3")] -> w761
            frame True {
            }
            frame False {
            }
          }
        }
        frame 18 {
          n302 = Decrement(x=w771) -> (x-1=w770:T21)
          n303 = Unbundle By Name(w770) -> ("Distance to DCS 2"=w769:i32)
          n304 = Less Or Equal To 0?(x=w769) -> (x <= 0?=w767:bool)
          n305 = case shown="True" w767 {
            tunnel: [u8 19 ("Det 3") u8 18 ("Det 3")] -> w768
            frame True {
            }
            frame False {
            }
          }
        }
        frame 19 {
          n306 = Decrement(x=w780) -> (x-1=w779:T21)
          n307 = Unbundle By Name(w779) -> ("Distance to DCS 2"=w778:i32)
          n308 = Add(x=w778, y=w777) -> (x+y=w776:i32)
          n309 = Less Or Equal To 0?(x=w776) -> (x <= 0?=w775:bool)
          n310 = case shown="True" w775 {
            tunnel: [u8 19 ("Det 3") w785] -> w782
            tunnel: w774 -> [_ w784]
            frame False {
            }
            frame True {
              n311 = case shown="True" w784 {
                tunnel: [_ u8 20 ("Det 3")] -> w785
                frame False {
                }
                frame True {
                }
              }
            }
          }
        }
        frame 20 {
          n312 = Decrement(x=w791) -> (x-1=w790:T21)
          n313 = Unbundle By Name(w790) -> ("Distance to front of LEIL Chamber"=w789:i32)
          n314 = Less Or Equal To 0?(x=w789) -> (x <= 0?=w787:bool)
          n315 = case shown="True" w787 {
            tunnel: [u8 21 ("Det 3") u8 20 ("Det 3")] -> w788
            frame True {
            }
            frame False {
            }
          }
        }
        frame 21 {
          n316 = Decrement(x=w800) -> (x-1=w799:T21)
          n317 = Unbundle By Name(w799) -> ("Distance to front of LEIL Chamber"=w798:i32)
          n318 = Add(x=w798, y=w797) -> (x+y=w796:i32)
          n319 = Less Or Equal To 0?(x=w796) -> (x <= 0?=w795:bool)
          n320 = case shown="True" w795 {
            tunnel: [u8 21 ("Det 3") _] -> w801
            frame False {
            }
            frame True {
            }
          }
        }
      }
      n321 = disable-structure shown="Disabled" {
        disable-tunnel: w239 -> [w301 w309]
        disable-tunnel: [w297 w308] -> w235
        disable-tunnel: [w299 _] -> w234
        disable-tunnel: w233 -> [w300 _]
        frame Disabled {
          n322 = case shown="1, Default" w301 {
            selector: w301 -> [_ w307]
            tunnel: [w304 w305] -> w298
            tunnel: w300 -> [w304 w306]
            frame 0 {
            }
            frame 1, Default {
              n323 = Max & Min(x=w307, y=w306) -> (min(x,y)=w305:i32)  [unwired: 1 out]
            }
          }
          n324 = Less Than 0?(x=w298) -> (x < 0?=w297:bool)
          n325 = case shown="False" w297 {
            tunnel: w298 -> [w303 _]
            tunnel: [w302 _] -> w299
            frame False {
              n326 = Decrement(x=w303) -> (x-1=w302:i32)
            }
            frame True {
            }
          }
        }
        frame Enabled {
          n327 = Not Equal To 0?(x=w309) -> (x != 0?=w308:bool)
        }
      }
      n328 = case shown="False" w229 {
        tunnel: [w286 w290] -> w228
        tunnel: w227 -> [_ w290]
        tunnel: [w284 w288] -> w226
        tunnel: w225 -> [w283 w288]
        tunnel: w224 -> [_ w289]
        tunnel: [w287 w289] -> w223
        tunnel: w222 -> [w287 _]
        tunnel: w221 -> [w285 _]
        tunnel: w220 -> [w286 _]
        frame False {
          n329 = To Fixed-Point(fixed-point type=w283, number=w285) -> (fixed-point=w284:fxp<+/-,64,-2>)
        }
        frame True {
        }
      }
      n330 = case shown="False" w235 {
        tunnel: w238 -> [_ w296]
        tunnel: [w291 w296] -> w237
        tunnel: w236 -> [w292 _]
        frame False {
          n331 = case shown="1, Default" w292 {
            selector: w292 -> [w293 w295]
            tunnel: [w293 w294] -> w291
            frame 0 {
            }
            frame 1, Default {
              n332 = Decrement(x=w295) -> (x-1=w294:u16)
            }
          }
        }
        frame True {
        }
      }
    }
    n333 = case shown="False" "Calibrate" {
      tunnel: w136 -> [w185 _]
      tunnel: w132 -> [w181 w211]
      tunnel: [w181 w209] -> w135
      tunnel: w134 -> [_ w210]
      frame False {
        n334 = local read "Particles Discarded"() -> (w183:i16)
        n335 = Not Equal To 0?(x=w185) -> (x != 0?=w184:bool[])
        n336 = Array To Cluster(array=w185) -> (cluster=w186:T22)
        n337 = Or Array Elements(Boolean array=w184) -> (logical OR=w182:bool)
        n338 = case shown="True" w182 {
          tunnel: w186 -> [_ w202]
          tunnel: w184 -> [_ w188]
          tunnel: w183 -> [_ w187]
          frame False {
          }
          frame True {
            n339 = local read "All Discard Points"() -> (w208:T4)
            n340 = Boolean To (0,1)(Boolean=w188) -> (0, 1=w189:i16[])
            n341 = Index Array(array=w189) -> (element #1=w191:i16, element #2=w192:i16, element #3=w193:i16, element #4=w194:i16, element #5=w195:i16, element #6=w196:i16, element #7=w197:i16, element #8=w198:i16, element #9=w199:i16, element #10=w200:i16, element #11=w190:i16)  [unwired: 11 in]
            n342 = Compound Arithmetic op=ADD(w191, w192, w193, w194, w195, w196, w197, w198, w199, w200, w190, w187) -> (→"Particles Discarded":i16)
            n343 = Cluster To Array(cluster=w208) -> (array=w204:T5[])
            n344 = Insert Into Array(array=w204, index=0, new element=w202) -> (w206:T5[])
            n345 = Delete From Array(array=w206) -> (array with subset deleted=w203:T5[])  [unwired: 2 in, 1 out]
            n346 = Array To Cluster(array=w203) -> (cluster=→"All Discard Points":T23)
          }
        }
      }
      frame True {
        n347 = for {
          tunnel: w210 -> [w214] mode=indexing
          tunnel: w211 -> [w213] mode=indexing
          tunnel: [w212] -> w209 mode=indexing
          n348 = Max & Min(x=w213, y=w214) -> (max(x,y)=w212:i32)  [unwired: 1 out]
        }
      }
    }
    n349 = Or Array Elements(Boolean array=w103) -> (logical OR=w97:bool)
    n350 = Array To Cluster(array=w94) -> (cluster=→"Velocity Count":T3)
    n351 = Array To Cluster(array=w93) -> (cluster=→"Mass":T2)
    n352 = Array To Cluster(array=w92) -> (cluster=→"Charge":T1)
    n353 = Bundle(w94, w93, w92) -> (w91:T24)  [unwired: 1 in]
    n354 = Not(x=w97) -> (.not. x?=w102:bool)
    n355 = Or Array Elements(Boolean array=w109) -> (logical OR=→"Plates":bool)
    n356 = Or Array Elements(Boolean array=w107) -> (logical OR=→"DCS 2":bool)
    n357 = Or Array Elements(Boolean array=w106) -> (logical OR=→"User Trigger":bool)
    n358 = Greater Than 0?(x=w124) -> (x > 0?=w123:bool[])
    n359 = And(x=w102, y=w100) -> (x .and. y?=w101:bool)
    n360 = Or Array Elements(Boolean array=w123) -> (logical OR=→"DCS 1":bool)
    n361 = local write "Armed"(w101) -> ()
  }
  n362 = while {
    stop <- FALSE stop-if-true
    w806 = TRUE ("IO Module\\PFI Enable")
    n363 = local read "DCS 2"() -> (w807:bool)
    n364 = local read "User Trigger"() -> (w805:bool)
    n365 = local read "DCS 1"() -> (w808:bool)
    n366 = local read "Plates"() -> (w809:bool)
    n367 = xnode "FPGA I/O Node"("IO Module\\PFI 0 Wr Data"=w809, "IO Module\\PFI 1 Wr Data"=w808, "IO Module\\PFI 2 Wr Data"=w807, "IO Module\\PFI 3 Wr Data"=w805) -> ()  [unwired: 4 in, 4 out]
    n368 = xnode "FPGA I/O Node"("IO Module\\PFI 0 WE"=w806, "IO Module\\PFI 1 WE"=w806, "IO Module\\PFI 2 WE"=w806, "IO Module\\PFI 3 WE"=w806) -> ()  [unwired: 4 in, 4 out]
  }
  n369 = node-c288(refnum<k21> "IO Module\\Data Clock" ("Source Name")) -> (w67:T12)
  n370 = timed-loop {
    timing: w67 -> [_]
    timing-out: [_] -> w66
    stop <- _ stop-if-true
    n371 = xnode "FPGA I/O Node"() -> ("IO Module\\AI 1"=w812:i16)  [unwired: 1 in, 1 out]
    n372 = xnode "FPGA I/O Node"() -> ("IO Module\\AI 0"=w813:i16)  [unwired: 1 in, 1 out]
    n373 = Bundle("IO Module\\AI 0"=w813, "IO Module\\AI 1"=w812) -> (→"Detectors":T25)  [unwired: 1 in]
  }
  n374 = node-c288(w66) -> ()
  n375 = node-c288(w63) -> ()
